vi "Vessel(FPGARef).vi"(8 "error in (no error)":errorcluster, 9 "FPGA VI Reference":refnum<k20>, 11 "UDP connection ID":refnum<k16>) -> (0 "error out":errorcluster, 3 "Vessel.lvclass":refnum<class "Vessel.lvclass">)   [LabVIEW 2014, in "Vessel.lvclass"]
uses:
  Vessel.lvclass
  Vessel().vi
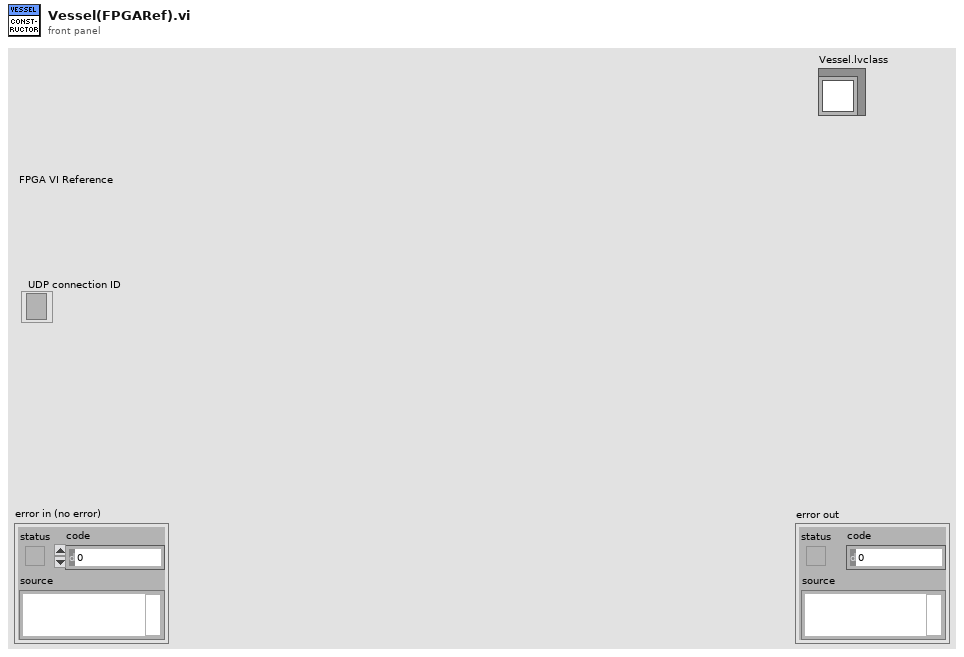
[diagram p1: front panel]
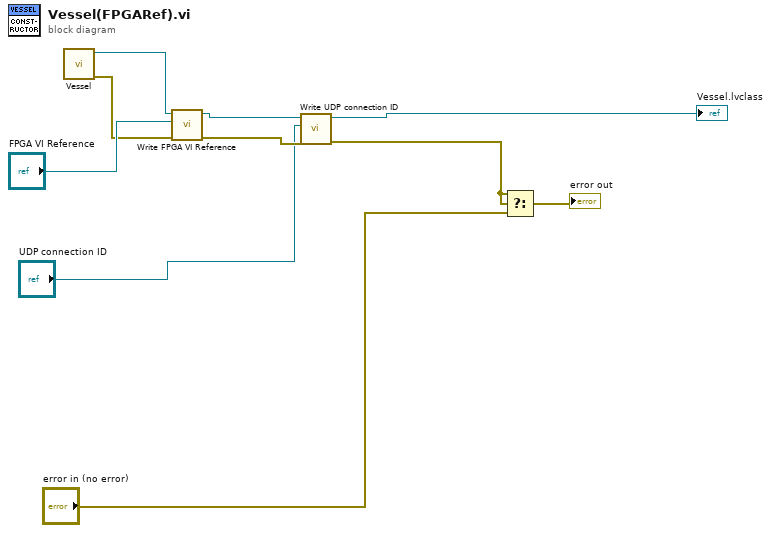
[diagram p0: block diagram]
diagram:
  n1 = call-poly "Vessel.vi"() -> ("error out"=w8:errorcluster, "Vessel.lvclass"=w9:refnum<class "Vessel.lvclass">)  [unwired: 10 in]
  n2 = call-dynamic "Write FPGA VI Reference.vi"("error in (no error)"=w8, "FPGA VI Reference Out 2"="FPGA VI Reference", "Vessel in"=w9) -> ("error out"=w5:errorcluster, "Vessel out"=w7:refnum<class "Vessel.lvclass">)  [unwired: 7 in]
  n3 = call-dynamic "Write UDP connection ID.vi"("error in (no error)"=w5, "UDP connection ID"="UDP connection ID", "Vessel in"=w7) -> ("error out"=w2:errorcluster, "Vessel out"=→"Vessel.lvclass":refnum<class "Vessel.lvclass">)  [unwired: 7 in]
  n4 = Select(t=w2, s=w2, f="error in (no error)") -> (s? t:f=→"error out":errorcluster)
